vi "Drinkindicator.vi"() -> (0 "water":u32, 1 "rum":u32, 2 "wisky":u32, 3 "coke":u32, 4 "sugar":u32, 5 "lime":u32, 6 "juice":u32)   [LabVIEW 2018]
uses:
  <vilib>/Utility/config.llb/Read Key (U32).vi
  <vilib>/Utility/config.llb/NI_LVConfig.lvlib
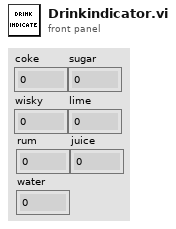
[diagram p1: front panel]
types:
  T1 = typedef "NI_LVConfig.lvlib/Config Data RefNum.ctl" = refnum<k1>
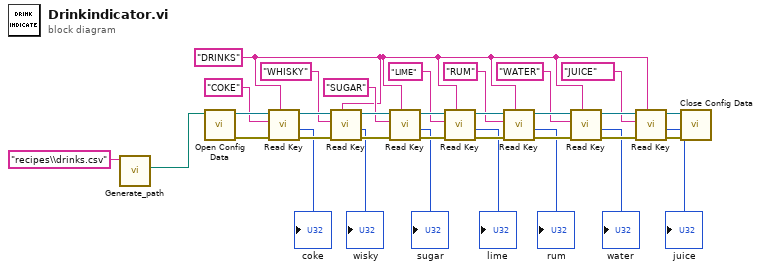
[diagram p0: block diagram]
diagram:
  w10 = "DRINKS"
  n1 = call "Generate_path.vi"("name or relative path"="recipes\\drinks.csv") -> ("MyFile"=w1:path)  [unwired: 10 in]
  n2 = call <vilib>:"Open Config Data.vi"("configuration file path"=w1) -> ("error out"=w25:errorcluster, "refnum"=w33:T1)  [unwired: 8 in, 1 out]
  n3 = call-poly <vilib>:"Read Key.vi"("section"=w10, "error in (no error)"=w25, "key"="COKE", "refnum"=w33) -> ("error out"=w24:errorcluster, "value"=→"coke":u32, "refnum out"=w32:T1)  [unwired: 4 in, 1 out]
  n4 = call-poly <vilib>:"Read Key.vi"("section"=w10, "error in (no error)"=w24, "key"="WHISKY", "refnum"=w32) -> ("error out"=w23:errorcluster, "value"=→"wisky":u32, "refnum out"=w31:T1)  [unwired: 4 in, 1 out]
  n5 = call-poly <vilib>:"Read Key.vi"("section"=w10, "error in (no error)"=w23, "key"="SUGAR", "refnum"=w31) -> ("error out"=w22:errorcluster, "value"=→"sugar":u32, "refnum out"=w30:T1)  [unwired: 4 in, 1 out]
  n6 = call-poly <vilib>:"Read Key.vi"("section"=w10, "error in (no error)"=w22, "key"="LIME", "refnum"=w30) -> ("error out"=w21:errorcluster, "value"=→"lime":u32, "refnum out"=w29:T1)  [unwired: 4 in, 1 out]
  n7 = call-poly <vilib>:"Read Key.vi"("section"=w10, "error in (no error)"=w21, "key"="RUM", "refnum"=w29) -> ("error out"=w20:errorcluster, "value"=→"rum":u32, "refnum out"=w28:T1)  [unwired: 4 in, 1 out]
  n8 = call-poly <vilib>:"Read Key.vi"("section"=w10, "error in (no error)"=w20, "key"="WATER", "refnum"=w28) -> ("error out"=w19:errorcluster, "value"=→"water":u32, "refnum out"=w27:T1)  [unwired: 4 in, 1 out]
  n9 = call-poly <vilib>:"Read Key.vi"("section"=w10, "error in (no error)"=w19, "key"="JUICE", "refnum"=w27) -> ("error out"=w18:errorcluster, "value"=→"juice":u32, "refnum out"=w26:T1)  [unwired: 4 in, 1 out]
  n10 = call <vilib>:"Close Config Data.vi"("error in (no error)"=w18, "refnum"=w26) -> ()  [unwired: 8 in, 2 out]
